vi "Part 2.vi"(11 "Input":string="Time:        40     81     77     72\nDistance:   219   1012   1365   1089") -> (3 "Output":i64)   [LabVIEW 2021]
uses:
  <userlib>/_OpenG.lib/string/string.llb/Convert EOLs (String)__ogtk.vi
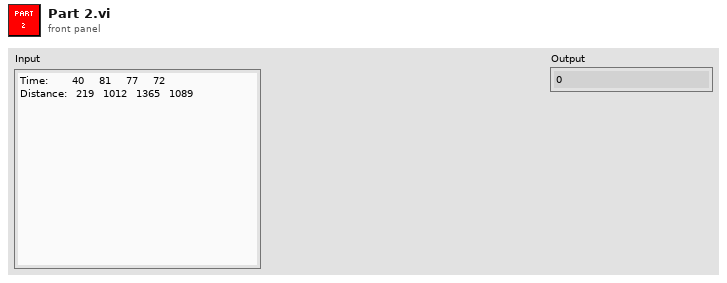
[diagram p1: front panel]
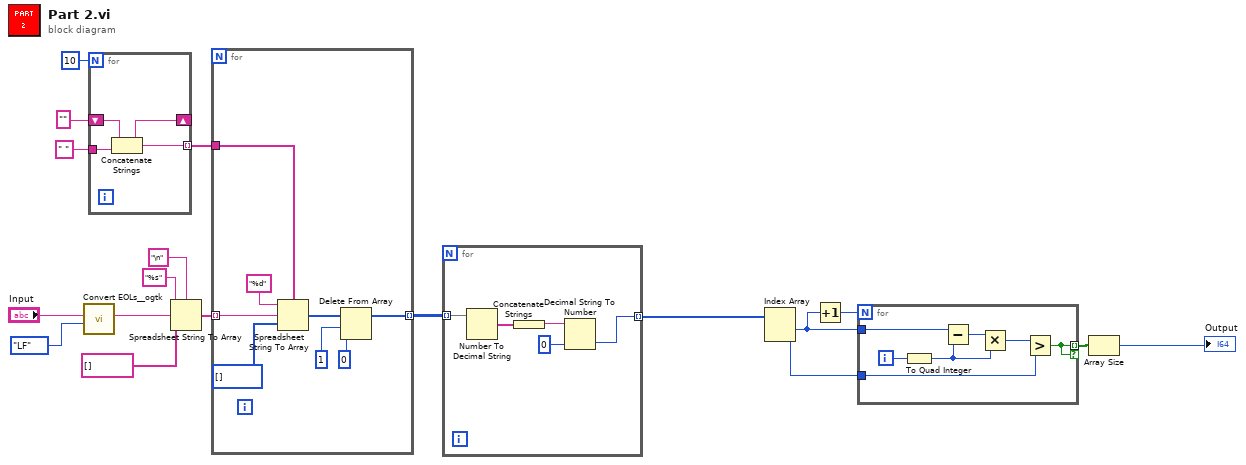
[diagram p0: block diagram]
diagram:
  n1 = call-poly <userlib>:"Convert EOLs__ogtk.vi"("Convert to:"=enum16{"CR", "LF", "CRLF"}."LF", "String in"="Input") -> ("String out"=w14:string)  [unwired: 9 in]
  n2 = for {
    N: 10 -> [_]
    tunnel: " " ("delimiter (Tab)") -> [w21]
    shift-right: [w19] -> _
    shift-left: "" -> [w20]
    tunnel: [w19] -> w8 mode=indexing
    n3 = Concatenate Strings(w20, w21) -> (w19:string)
  }
  n4 = Spreadsheet String To Array(delimiter (Tab)="\n", format string="%s", spreadsheet string=w14, array type (2D Dbl)=string[] []) -> (array=w12:string[])
  n5 = for {
    tunnel: w12 -> [w28] mode=indexing
    tunnel: w8 -> [w29]
    tunnel: [w24] -> w7 mode=indexing
    n6 = Spreadsheet String To Array(delimiter (Tab)=w29, format string="%d", spreadsheet string=w28, array type (2D Dbl)=i64[] []) -> (array=w25:i64[])
    n7 = Delete From Array(array=w25, length=1 ("index"), index=0) -> (array with subset deleted=w24:i64[])  [unwired: 1 out]
  }
  n8 = for {
    tunnel: w7 -> [w34] mode=indexing
    tunnel: [w31] -> w6 mode=indexing
    n9 = Number To Decimal String(number=w34) -> (decimal integer string=w33:string[])  [unwired: 1 in]
    n10 = Concatenate Strings(w33) -> (w32:string)
    n11 = Decimal String To Number(string=w32, default (0L)=i64 0) -> (number=w31:i64)  [unwired: 1 in, 1 out]
  }
  n12 = Index Array(array=w6) -> (element #1=w3:i64, element #2=w4:i64)  [unwired: 2 in]
  n13 = Increment(x=w3) -> (x+1=w5:i64)
  n14 = for {
    N: w5 -> [_]
    tunnel: w4 -> [w37]
    tunnel: w3 -> [w41]
    tunnel: [w35] -> w2 mode=indexing if=w35
    i -> [w39]
    n15 = To Quad Integer(1:w39) -> (0:w36:i64)
    n16 = Subtract(x=w41, y=w36) -> (x-y=w40:i64)
    n17 = Multiply(x=w40, y=w36) -> (x*y=w38:i64)
    n18 = Greater?(x=w38, y=w37) -> (0:w35:bool)
  }
  n19 = Array Size(array=w2) -> (size(s)=→"Output":i32)
